vi "ConvertStatusRegisterToSystemStatus.vi"(0 "Status":T2, 5 "error in":errorcluster) -> (14 "SystemStatus":T1, 19 "error out":errorcluster)   [LabVIEW 2020]
uses:
  Status.ctl
  SystemStatus.ctl
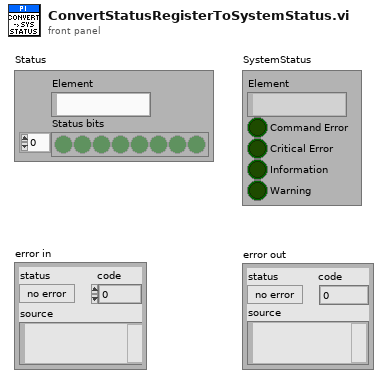
[diagram p1: front panel]
types:
  T1 = typedef "SystemStatus.ctl" = cluster{"Element":string, "Command Error":bool, "Critical Error":bool, "Information":bool, "Warning":bool}
  T2 = typedef "Status.ctl" = cluster{"Element":string, "Status bits":bool[]}
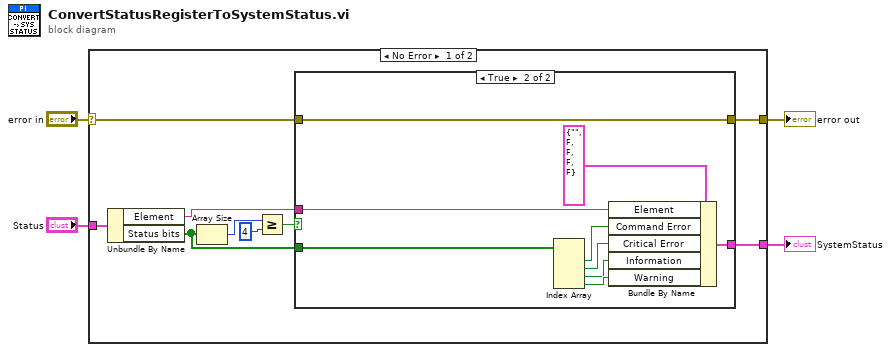
[diagram p0: block diagram]
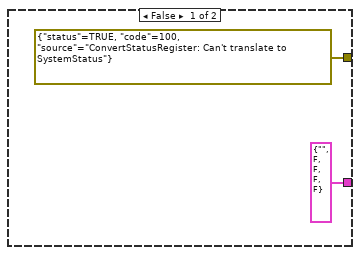
[diagram p2: hidden frame]
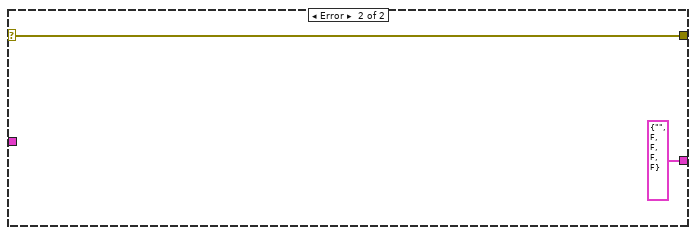
[diagram p3: hidden frame]
diagram:
  n1 = case shown="No Error" "error in" {
    selector: "error in" -> [w6 w26]
    tunnel: [w5 w26] -> w3
    tunnel: "Status" -> [w13 _]
    tunnel: [w7 T1 {"Element"="", "Command Error"=FALSE, "Critical Error"=FALSE, "Information"=FALSE, "Warning"=FALSE} ("SystemStatus")] -> w1
    frame No Error {
      n2 = Unbundle By Name(w13) -> ("Element"=w10:string, "Status bits"=w8:bool[])
      n3 = Array Size(array=w8) -> (size(s)=w11:i32)
      n4 = Greater Or Equal?(x=w11, y=4) -> (x >= y?=w12:bool)
      n5 = case shown="True" w12 {
        tunnel: w10 -> [_ w19]
        tunnel: w8 -> [_ w18]
        tunnel: [T1 {"Element"="", "Command Error"=FALSE, "Critical Error"=FALSE, "Information"=FALSE, "Warning"=FALSE} ("SystemStatus") w17] -> w7
        tunnel: w6 -> [_ w16]
        tunnel: [errorcluster {"status"=TRUE, "code"=100, "source"="ConvertStatusRegister: Can't translate to SystemStatus"} ("error out") w16] -> w5
        frame False {
        }
        frame True {
          n6 = Index Array(array=w18) -> (element #1=w21:bool, element #2=w22:bool, element #3=w23:bool, element #4=w24:bool)  [unwired: 4 in]
          n7 = Bundle By Name(cluster=T1 {"Element"="", "Command Error"=FALSE, "Critical Error"=FALSE, "Information"=FALSE, "Warning"=FALSE} ("SystemStatus"), "Element"=w19, "Command Error"=w21, "Critical Error"=w22, "Information"=w23, "Warning"=w24) -> (w17:T1)
        }
      }
    }
    frame Error {
    }
  }
  "error out" <- w3
  "SystemStatus" <- w1
